vi "Make Config File Information.vi"(0 "VISA resource name":refnum<visa-resource-name>, 5 "Command (\"\")":string, 11 "error in (no error)":errorcluster) -> (4 "VISA resource name out":refnum<visa-resource-name>, 6 "Result":string, 15 "error out":errorcluster)   [LabVIEW 2020, in "Yokogawa GX Series.lvlib"]
doc: "Returns result of communication command."
uses:
  <instrlib>/Yokogawa GX Series/Yokogawa GX Series.lvlib
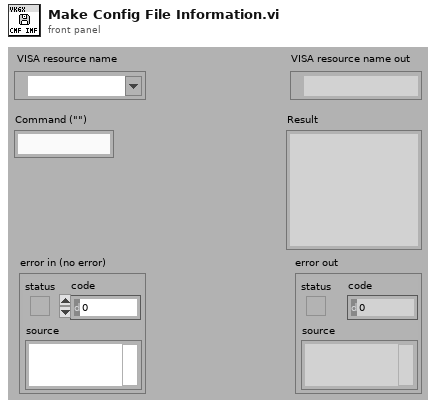
[diagram p1: front panel]
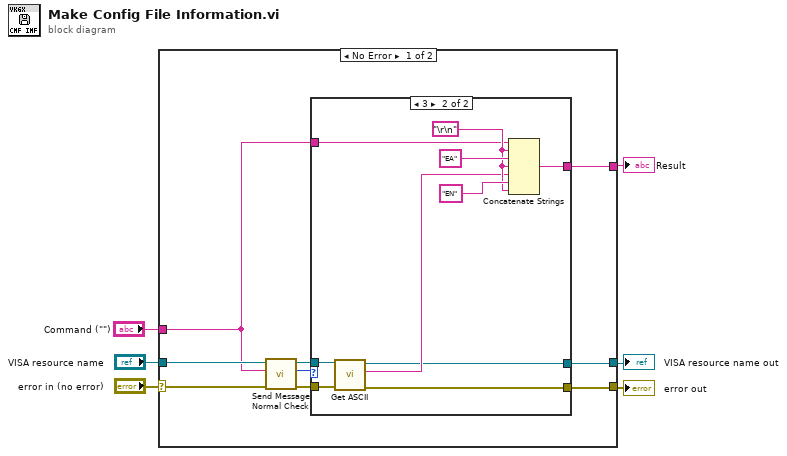
[diagram p0: block diagram]
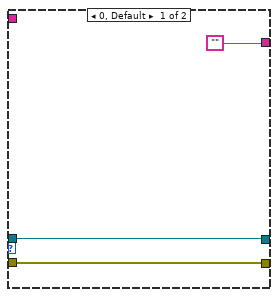
[diagram p2: hidden frame]
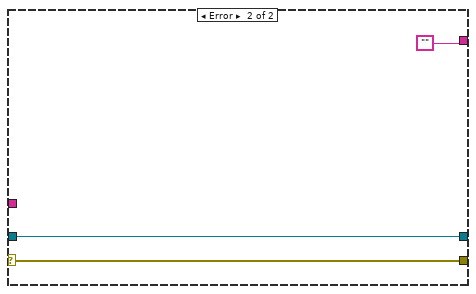
[diagram p3: hidden frame]
diagram:
  n1 = case shown="No Error" "error in (no error)" {
    selector: "error in (no error)" -> [w11 w30]
    tunnel: [w15 w31] -> w6
    tunnel: [w14 w30] -> w5
    tunnel: "VISA resource name" -> [w13 w31]
    tunnel: "Command (\"\")" -> [w10 _]
    tunnel: [w12 ""] -> w2
    frame No Error {
      n2 = call <instrlib>:"Send Message Normal Check.vi"("error in (no error)"=w11, "Send Message (\"\")"=w10, "VISA resource name"=w13) -> ("error out"=w8:errorcluster, "Response Type"=w7:i32, "VISA resource name out"=w9:refnum<visa-resource-name>)  [unwired: 3 in, 3 out]
      n3 = case shown="3" w7 {
        tunnel: w10 -> [_ w25]
        tunnel: w9 -> [w18 w24]
        tunnel: w8 -> [w17 w23]
        tunnel: [w18 w21] -> w15
        tunnel: [w17 w20] -> w14
        tunnel: ["" w19] -> w12
        frame 0, Default {
        }
        frame 3 {
          w26 = "\r\n"
          n4 = call <instrlib>:"Get ASCII.vi"("error in (no error)"=w23, "VISA resource name"=w24) -> ("error out"=w20:errorcluster, "ASCII Data"=w22:string, "VISA resource name out"=w21:refnum<visa-resource-name>)  [unwired: 7 in]
          n5 = Concatenate Strings(w25, w26, "EA", w26, w22, "EN", w26) -> (w19:string)
        }
      }
    }
    frame Error {
    }
  }
  "error out" <- w5
  "VISA resource name out" <- w6
  "Result" <- w2
